vi "Host Port.vi"(11 "URI in":refnum<class "URI.lvclass">) -> (2 "Port":u16, 3 "Host":u32, 5 "Port Unset":bool)   [LabVIEW 2020, in "URI.lvlib" / "URI.lvclass"]
uses:
  URI.lvclass
  URI.lvclass/URI.ctl
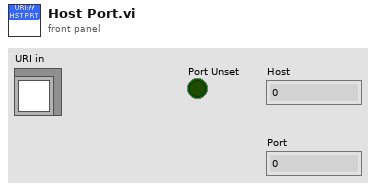
[diagram p1: front panel]
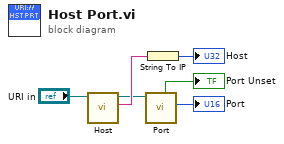
[diagram p0: block diagram]
diagram:
  n1 = call "Host.vi"("URI in"="URI in") -> ("Host"=w5:string, "URI out"=w3:refnum<class "URI.lvclass">)  [unwired: 9 in]
  n2 = call "Port.vi"("URI in"=w3) -> ("Port"=→"Port":u16, "Unset"=→"Port Unset":bool)  [unwired: 8 in, 1 out]
  n3 = String To IP(1:w5) -> (0:→"Host":u32)
